vi "VISJS Viewer.vi"(4 "Extra Scripts":string, 5 "FileDependency In":map{path, T1}(c390), 6 "Options":string, 7 "OpenWebBrowser(False)":bool, 8 "error in":errorcluster, 9 "Embedd VISJS Librarya in HTMl File(False)":bool, 10 "HTMLFilePath":path, 11 "LibraryDependency":map{path, T3}(c390)) -> (0 "error out":errorcluster, 3 "HTMLFileContent":string)   [LabVIEW 2020, in "VISJS Viewer.lvlib"] (continued)
function(){if(\"undefined\"==typeof Reflect||!MT)return!1;if(MT.sham)return!1;if(\"function\"==typeof Proxy)return!0;try{return Boolean.prototype.valueOf.call(MT(Boolean,[],(function(){}))),!0}catch(g){return!1}}();return function(){var A,e=nb(g);if(t){var C=nb(this).constructor;A=MT(e,arguments,C)}else A=e.apply(this,arguments);return Ib(this,A)}}var NR=function(g){Cb(A,g);var t=DR(A);function A(g,e,C){return cn(this,A),t.call(this,g,e,C)}return kd(A,[{key:\"_line\",value:function(g,t,A){this._bezierCurve(g,t,A)}},{key:\"getViaNode\",value:function(){return this._getViaCoordinates()}},{key:\"_getViaCoordinates\",value:function(){var g,t,A=this.options.smooth.roundness,e=this.options.smooth.type,C=Math.abs(this.from.x-this.to.x),I=Math.abs(this.from.y-this.to.y);if(\"discrete\"===e||\"diagonalCross\"===e){var i,o;i=o=C<=I?A*I:A*C,this.from.x>this.to.x&&(i=-i),this.from.y>=this.to.y&&(o=-o);var n=this.from.x+i,r=this.from.y+o;return\"discrete\"===e&&(C<=I?n=C<A*I?this.from.x:n:r=I<A*C?this.from.y:r),{x:n,y:r}}if(\"straightCross\"===e){var s=(1-A)*C,a=(1-A)*I;return C<=I?(s=0,this.from.y<this.to.y&&(a=-a)):(this.from.x<this.to.x&&(s=-s),a=0),{x:this.to.x+s,y:this.to.y+a}}if(\"horizontal\"===e){var d=(1-A)*C;return this.from.x<this.to.x&&(d=-d),{x:this.to.x+d,y:this.from.y}}if(\"vertical\"===e){var h=(1-A)*I;return this.from.y<this.to.y&&(h=-h),{x:this.from.x,y:this.to.y+h}}if(\"curvedCW\"===e){C=this.to.x-this.from.x,I=this.from.y-this.to.y;var l=Math.sqrt(C*C+I*I),c=Math.PI,u=(Math.atan2(I,C)+(.5*A+.5)*c)%(2*c);return{x:this.from.x+(.5*A+.5)*l*Math.sin(u),y:this.from.y+(.5*A+.5)*l*Math.cos(u)}}if(\"curvedCCW\"===e){C=this.to.x-this.from.x,I=this.from.y-this.to.y;var p=Math.sqrt(C*C+I*I),f=Math.PI,v=(Math.atan2(I,C)+(.5*-A+.5)*f)%(2*f);return{x:this.from.x+(.5*A+.5)*p*Math.sin(v),y:this.from.y+(.5*A+.5)*p*Math.cos(v)}}g=t=C<=I?A*I:A*C,this.from.x>this.to.x&&(g=-g),this.from.y>=this.to.y&&(t=-t);var y=this.from.x+g,m=this.from.y+t;return C<=I?y=this.from.x<=this.to.x?this.to.x<y?this.to.x:y:this.to.x>y?this.to.x:y:m=this.from.y>=this.to.y?this.to.y>m?this.to.y:m:this.to.y<m?this.to.y:m,{x:y,y:m}}},{key:\"_findBorderPosition\",value:function(g,t){var A=arguments.length>2&&void 0!==arguments[2]?arguments[2]:{};return this._findBorderPositionBezier(g,t,A.via)}},{key:\"_getDistanceToEdge\",value:function(g,t,A,e,C,I){var i=arguments.length>6&&void 0!==arguments[6]?arguments[6]:this._getViaCoordinates();return this._getDistanceToBezierEdge(g,t,A,e,C,I,i)}},{key:\"getPoint\",value:function(g){var t=arguments.length>1&&void 0!==arguments[1]?arguments[1]:this._getViaCoordinates(),A=g;return{x:Math.pow(1-A,2)*this.fromPoint.x+2*A*(1-A)*t.x+Math.pow(A,2)*this.toPoint.x,y:Math.pow(1-A,2)*this.fromPoint.y+2*A*(1-A)*t.y+Math.pow(A,2)*this.toPoint.y}}}]),A}(ER);function RR(g){var t=function(){if(\"undefined\"==typeof Reflect||!MT)return!1;if(MT.sham)return!1;if(\"function\"==typeof Proxy)return!0;try{return Boolean.prototype.valueOf.call(MT(Boolean,[],(function(){}))),!0}catch(g){return!1}}();return function(){var A,e=nb(g);if(t){var C=nb(this).constructor;A=MT(e,arguments,C)}else A=e.apply(this,arguments);return Ib(this,A)}}var PR=function(g){Cb(A,g);var t=RR(A);function A(g,e,C){return cn(this,A),t.call(this,g,e,C)}return kd(A,[{key:\"_getDistanceToBezierEdge2\",value:function(g,t,A,e,C,I,i,o){for(var n=1e9,r=g,s=t,a=[0,0,0,0],d=1;d<10;d++){var h=.1*d;a[0]=Math.pow(1-h,3),a[1]=3*h*Math.pow(1-h,2),a[2]=3*Math.pow(h,2)*(1-h),a[3]=Math.pow(h,3);var l=a[0]*g+a[1]*i.x+a[2]*o.x+a[3]*A,c=a[0]*t+a[1]*i.y+a[2]*o.y+a[3]*e;if(d>0){var u=this._getDistanceToLine(r,s,l,c,C,I);n=u<n?u:n}r=l,s=c}return n}}]),A}(ER);function MR(g){var t=function(){if(\"undefined\"==typeof Reflect||!MT)return!1;if(MT.sham)return!1;if(\"function\"==typeof Proxy)return!0;try{return Boolean.prototype.valueOf.call(MT(Boolean,[],(function(){}))),!0}catch(g){return!1}}();return function(){var A,e=nb(g);if(t){var C=nb(this).constructor;A=MT(e,arguments,C)}else A=e.apply(this,arguments);return Ib(this,A)}}var BR=function(g){Cb(A,g);var t=MR(A);function A(g,e,C){return cn(this,A),t.call(this,g,e,C)}return kd(A,[{key:\"_line\",value:function(g,t,A){var e=A[0],C=A[1];this._bezierCurve(g,t,e,C)}},{key:\"_getViaCoordinates\",value:function(){var g,t,A,e,C=this.from.x-this.to.x,I=this.from.y-this.to.y,i=this.options.smooth.roundness;return(Math.abs(C)>Math.abs(I)||!0===this.options.smooth.forceDirection||\"horizontal\"===this.options.smooth.forceDirection)&&\"vertical\"!==this.options.smooth.forceDirection?(t=this.from.y,e=this.to.y,g=this.from.x-i*C,A=this.to.x+i*C):(t=this.from.y-i*I,e=this.to.y+i*I,g=this.from.x,A=this.to.x),[{x:g,y:t},{x:A,y:e}]}},{key:\"getViaNode\",value:function(){return this._getViaCoordinates()}},{key:\"_findBorderPosition\",value:function(g,t){return this._findBorderPositionBezier(g,t)}},{key:\"_getDistanceToEdge\",value:function(g,t,A,e,C,I){var i=lh(arguments.length>6&&void 0!==arguments[6]?arguments[6]:this._getViaCoordinates(),2),o=i[0],n=i[1];return this._getDistanceToBezierEdge2(g,t,A,e,C,I,o,n)}},{key:\"getPoint\",value:function(g){var t=lh(arguments.length>1&&void 0!==arguments[1]?arguments[1]:this._getViaCoordinates(),2),A=t[0],e=t[1],C=g,I=[Math.pow(1-C,3),3*C*Math.pow(1-C,2),3*Math.pow(C,2)*(1-C),Math.pow(C,3)];return{x:I[0]*this.fromPoint.x+I[1]*A.x+I[2]*e.x+I[3]*this.toPoint.x,y:I[0]*this.fromPoint.y+I[1]*A.y+I[2]*e.y+I[3]*this.toPoint.y}}}]),A}(PR);function zR(g){var t=function(){if(\"undefined\"==typeof Reflect||!MT)return!1;if(MT.sham)return!1;if(\"function\"==typeof Proxy)return!0;try{return Boolean.prototype.valueOf.call(MT(Boolean,[],(function(){}))),!0}catch(g){return!1}}();return function(){var A,e=nb(g);if(t){var C=nb(this).constructor;A=MT(e,arguments,C)}else A=e.apply(this,arguments);return Ib(this,A)}}var SR=function(g){Cb(A,g);var t=zR(A);function A(g,e,C){return cn(this,A),t.call(this,g,e,C)}return kd(A,[{key:\"_line\",value:function(g,t){g.beginPath(),g.moveTo(this.fromPoint.x,this.fromPoint.y),g.lineTo(this.toPoint.x,this.toPoint.y),this.enableShadow(g,t),g.stroke(),this.disableShadow(g,t)}},{key:\"getViaNode\",value:function(){}},{key:\"getPoint\",value:function(g){return{x:(1-g)*this.fromPoint.x+g*this.toPoint.x,y:(1-g)*this.fromPoint.y+g*this.toPoint.y}}},{key:\"_findBorderPosition\",value:function(g,t){var A=this.to,e=this.from;g.id===this.from.id&&(A=this.from,e=this.to);var C=Math.atan2(A.y-e.y,A.x-e.x),I=A.x-e.x,i=A.y-e.y,o=Math.sqrt(I*I+i*i),n=(o-g.distanceToBorder(t,C))/o;return{x:(1-n)*e.x+n*A.x,y:(1-n)*e.y+n*A.y,t:0}}},{key:\"_getDistanceToEdge\",value:function(g,t,A,e,C,I){return this._getDistanceToLine(g,t,A,e,C,I)}}]),A}(bR),ZR=function(){function g(t,A,e,C,I){if(cn(this,g),void 0===A)throw new Error(\"No body provided\");this.options=av(C),this.globalOptions=C,this.defaultOptions=I,this.body=A,this.imagelist=e,this.id=void 0,this.fromId=void 0,this.toId=void 0,this.selected=!1,this.hover=!1,this.labelDirty=!0,this.baseWidth=this.options.width,this.baseFontSize=this.options.font.size,this.from=void 0,this.to=void 0,this.edgeType=void 0,this.connected=!1,this.labelModule=new qD(this.body,this.options,!0),this.setOptions(t)}return kd(g,[{key:\"setOptions\",value:function(t){if(t){var A=void 0!==t.physics&&this.options.physics!==t.physics||void 0!==t.hidden&&(this.options.hidden||!1)!==(t.hidden||!1)||void 0!==t.from&&this.options.from!==t.from||void 0!==t.to&&this.options.to!==t.to;g.parseOptions(this.options,t,!0,this.globalOptions),void 0!==t.id&&(this.id=t.id),void 0!==t.from&&(this.fromId=t.from),void 0!==t.to&&(this.toId=t.to),void 0!==t.title&&(this.title=t.title),void 0!==t.value&&(t.value=SD(t.value));var e=[t,this.options,this.defaultOptions];return this.chooser=YD(\"edge\",e),this.updateLabelModule(t),A=this.updateEdgeType()||A,this._setInteractionWidths(),this.connect(),A}}},{key:\"getFormattingValues\",value:function(){var g=!0===this.options.arrows.to||!0===this.options.arrows.to.enabled,t=!0===this.options.arrows.from||!0===this.options.arrows.from.enabled,A=!0===this.options.arrows.middle||!0===this.options.arrows.middle.enabled,e=this.options.color.inherit,C={toArrow:g,toArrowScale:this.options.arrows.to.scaleFactor,toArrowType:this.options.arrows.to.type,toArrowSrc:this.options.arrows.to.src,toArrowImageWidth:this.options.arrows.to.imageWidth,toArrowImageHeight:this.options.arrows.to.imageHeight,middleArrow:A,middleArrowScale:this.options.arrows.middle.scaleFactor,middleArrowType:this.options.arrows.middle.type,middleArrowSrc:this.options.arrows.middle.src,middleArrowImageWidth:this.options.arrows.middle.imageWidth,middleArrowImageHeight:this.options.arrows.middle.imageHeight,fromArrow:t,fromArrowScale:this.options.arrows.from.scaleFactor,fromArrowType:this.options.arrows.from.type,fromArrowSrc:this.options.arrows.from.src,fromArrowImageWidth:this.options.arrows.from.imageWidth,fromArrowImageHeight:this.options.arrows.from.imageHeight,arrowStrikethrough:this.options.arrowStrikethrough,color:e?void 0:this.options.color.color,inheritsColor:e,opacity:this.options.color.opacity,hidden:this.options.hidden,length:this.options.length,shadow:this.options.shadow.enabled,shadowColor:this.options.shadow.color,shadowSize:this.options.shadow.size,shadowX:this.options.shadow.x,shadowY:this.options.shadow.y,dashes:this.options.dashes,width:this.options.width,background:this.options.background.enabled,backgroundColor:this.options.background.color,backgroundSize:this.options.background.size,backgroundDashes:this.options.background.dashes};if(this.selected||this.hover)if(!0===this.chooser){if(this.selected){var I=this.options.selectionWidth;\"function\"==typeof I?C.width=I(C.width):\"number\"==typeof I&&(C.width+=I),C.width=Math.max(C.width,.3/this.body.view.scale),C.color=this.options.color.highlight,C.shadow=this.options.shadow.enabled}else if(this.hover){var i=this.options.hoverWidth;\"function\"==typeof i?C.width=i(C.width):\"number\"==typeof i&&(C.width+=i),C.width=Math.max(C.width,.3/this.body.view.scale),C.color=this.options.color.hover,C.shadow=this.options.shadow.enabled}}else\"function\"==typeof this.chooser&&(this.chooser(C,this.options.id,this.selected,this.hover),void 0!==C.color&&(C.inheritsColor=!1),!1===C.shadow&&(C.shadowColor===this.options.shadow.color&&C.shadowSize===this.options.shadow.size&&C.shadowX===this.options.shadow.x&&C.shadowY===this.options.shadow.y||(C.shadow=!0)));else C.shadow=this.options.shadow.enabled,C.width=Math.max(C.width,.3/this.body.view.scale);return C}},{key:\"updateLabelModule\",value:function(g){var t=[g,this.options,this.globalOptions,this.defaultOptions];this.labelModule.update(this.options,t),void 0!==this.labelModule.baseSize&&(this.baseFontSize=this.labelModule.baseSize)}},{key:\"updateEdgeType\",value:function(){var g=this.options.smooth,t=!1,A=!0;return void 0!==this.edgeType&&((this.edgeType instanceof TR&&!0===g.enabled&&\"dynamic\"===g.type||this.edgeType instanceof BR&&!0===g.enabled&&\"cubicBezier\"===g.type||this.edgeType instanceof NR&&!0===g.enabled&&\"dynamic\"!==g.type&&\"cubicBezier\"!==g.type||this.edgeType instanceof SR&&!1===g.type.enabled)&&(A=!1),!0===A&&(t=this.cleanup())),!0===A?!0===g.enabled?\"dynamic\"===g.type?(t=!0,this.edgeType=new TR(this.options,this.body,this.labelModule)):\"cubicBezier\"===g.type?this.edgeType=new BR(this.options,this.body,this.labelModule):this.edgeType=new NR(this.options,this.body,this.labelModule):this.edgeType=new SR(this.options,this.body,this.labelModule):this.edgeType.setOptions(this.options),t}},{key:\"connect\",value:function(){this.disconnect(),this.from=this.body.nodes[this.fromId]||void 0,this.to=this.body.nodes[this.toId]||void 0,this.connected=void 0!==this.from&&void 0!==this.to,!0===this.connected?(this.from.attachEdge(this),this.to.attachEdge(this)):(this.from&&this.from.detachEdge(this),this.to&&this.to.detachEdge(this)),this.edgeType.connect()}},{key:\"disconnect\",value:function(){this.from&&(this.from.detachEdge(this),this.from=void 0),this.to&&(this.to.detachEdge(this),this.to=void 0),this.connected=!1}},{key:\"getTitle\",value:function(){return this.title}},{key:\"isSelected\",value:function(){return this.selected}},{key:\"getValue\",value:function(){return this.options.value}},{key:\"setValueRange\",value:function(g,t,A){if(void 0!==this.options.value){var e=this.options.scaling.customScalingFunction(g,t,A,this.options.value),C=this.options.scaling.max-this.options.scaling.min;if(!0===this.options.scaling.label.enabled){var I=this.options.scaling.label.max-this.options.scaling.label.min;this.options.font.size=this.options.scaling.label.min+e*I}this.options.width=this.options.scaling.min+e*C}else this.options.width=this.baseWidth,this.options.font.size=this.baseFontSize;this._setInteractionWidths(),this.updateLabelModule()}},{key:\"_setInteractionWidths\",value:function(){\"function\"==typeof this.options.hoverWidth?this.edgeType.hoverWidth=this.options.hoverWidth(this.options.width):this.edgeType.hoverWidth=this.options.hoverWidth+this.options.width,\"function\"==typeof this.options.selectionWidth?this.edgeType.selectionWidth=this.options.selectionWidth(this.options.width):this.edgeType.selectionWidth=this.options.selectionWidth+this.options.width}},{key:\"draw\",value:function(g){var t=this.getFormattingValues();if(!t.hidden){var A=this.edgeType.getViaNode();this.edgeType.drawLine(g,t,this.selected,this.hover,A),this.drawLabel(g,A)}}},{key:\"drawArrows\",value:function(g){var t=this.getFormattingValues();if(!t.hidden){var A=this.edgeType.getViaNode(),e={};this.edgeType.fromPoint=this.edgeType.from,this.edgeType.toPoint=this.edgeType.to,t.fromArrow&&(e.from=this.edgeType.getArrowData(g,\"from\",A,this.selected,this.hover,t),!1===t.arrowStrikethrough&&(this.edgeType.fromPoint=e.from.core),t.fromArrowSrc&&(e.from.image=this.imagelist.load(t.fromArrowSrc)),t.fromArrowImageWidth&&(e.from.imageWidth=t.fromArrowImageWidth),t.fromArrowImageHeight&&(e.from.imageHeight=t.fromArrowImageHeight)),t.toArrow&&(e.to=this.edgeType.getArrowData(g,\"to\",A,this.selected,this.hover,t),!1===t.arrowStrikethrough&&(this.edgeType.toPoint=e.to.core),t.toArrowSrc&&(e.to.image=this.imagelist.load(t.toArrowSrc)),t.toArrowImageWidth&&(e.to.imageWidth=t.toArrowImageWidth),t.toArrowImageHeight&&(e.to.imageHeight=t.toArrowImageHeight)),t.middleArrow&&(e.middle=this.edgeType.getArrowData(g,\"middle\",A,this.selected,this.hover,t),t.middleArrowSrc&&(e.middle.image=this.imagelist.load(t.middleArrowSrc)),t.middleArrowImageWidth&&(e.middle.imageWidth=t.middleArrowImageWidth),t.middleArrowImageHeight&&(e.middle.imageHeight=t.middleArrowImageHeight)),t.fromArrow&&this.edgeType.drawArrowHead(g,t,this.selected,this.hover,e.from),t.middleArrow&&this.edgeType.drawArrowHead(g,t,this.selected,this.hover,e.middle),t.toArrow&&this.edgeType.drawArrowHead(g,t,this.selected,this.hover,e.to)}}},{key:\"drawLabel\",value:function(g,t){if(void 0!==this.options.label){var A,e=this.from,C=this.to;if(this.labelModule.differentState(this.selected,this.hover)&&this.labelModule.getTextSize(g,this.selected,this.hover),e.id!=C.id){this.labelModule.pointToSelf=!1,A=this.edgeType.getPoint(.5,t),g.save();var I=this._getRotation(g);0!=I.angle&&(g.translate(I.x,I.y),g.rotate(I.angle)),this.labelModule.draw(g,A.x,A.y,this.selected,this.hover),g.restore()}else{this.labelModule.pointToSelf=!0;var i=UD(g,this.options.selfReference.angle,this.options.selfReference.size,e);A=this._pointOnCircle(i.x,i.y,this.options.selfReference.size,this.options.selfReference.angle),this.labelModule.draw(g,A.x,A.y,this.selected,this.hover)}}}},{key:\"getItemsOnPoint\",value:function(g){var t=[];if(this.labelModule.visible()){var A=this._getRotation();WD(this.labelModule.getSize(),g,A)&&t.push({edgeId:this.id,labelId:0})}var e={left:g.x,top:g.y};return this.isOverlappingWith(e)&&t.push({edgeId:this.id}),t}},{key:\"isOverlappingWith\",value:function(g){if(this.connected){var t=this.from.x,A=this.from.y,e=this.to.x,C=this.to.y,I=g.left,i=g.top;return this.edgeType.getDistanceToEdge(t,A,e,C,I,i)<10}return!1}},{key:\"_getRotation\",value:function(g){var t=this.edgeType.getViaNode(),A=this.edgeType.getPoint(.5,t);void 0!==g&&this.labelModule.calculateLabelSize(g,this.selected,this.hover,A.x,A.y);var e={x:A.x,y:this.labelModule.size.yLine,angle:0};if(!this.labelModule.visible())return e;if(\"horizontal\"===this.options.font.align)return e;var C=this.from.y-this.to.y,I=this.from.x-this.to.x,i=Math.atan2(C,I);return(i<-1&&I<0||i>0&&I<0)&&(i+=Math.PI),e.angle=i,e}},{key:\"_pointOnCircle\",value:function(g,t,A,e){return{x:g+A*Math.cos(e),y:t-A*Math.sin(e)}}},{key:\"select\",value:function(){this.selected=!0}},{key:\"unselect\",value:function(){this.selected=!1}},{key:\"cleanup\",value:function(){return this.edgeType.cleanup()}},{key:\"remove\",value:function(){this.cleanup(),this.disconnect(),delete this.body.edges[this.id]}},{key:\"endPointsValid\",value:function(){return void 0!==this.body.nodes[this.fromId]&&void 0!==this.body.nodes[this.toId]}}],[{key:\"parseOptions\",value:function(g,t){var A=arguments.length>2&&void 0!==arguments[2]&&arguments[2],e=arguments.length>3&&void 0!==arguments[3]?arguments[3]:{},C=arguments.length>4&&void 0!==arguments[4]&&arguments[4];if(Xf([\"endPointOffset\",\"arrowStrikethrough\",\"id\",\"from\",\"hidden\",\"hoverWidth\",\"labelHighlightBold\",\"length\",\"line\",\"opacity\",\"physics\",\"scaling\",\"selectionWidth\",\"selfReferenceSize\",\"selfReference\",\"to\",\"title\",\"value\",\"width\",\"font\",\"chosen\",\"widthConstraint\"],g,t,A),void 0!==t.endPointOffset&&void 0!==t.endPointOffset.from&&(Ym(t.endPointOffset.from)?g.endPointOffset.from=t.endPointOffset.from:(g.endPointOffset.from=void 0!==e.endPointOffset.from?e.endPointOffset.from:0,console.error(\"endPointOffset.from is not a valid number\"))),void 0!==t.endPointOffset&&void 0!==t.endPointOffset.to&&(Ym(t.endPointOffset.to)?g.endPointOffset.to=t.endPointOffset.to:(g.endPointOffset.to=void 0!==e.endPointOffset.to?e.endPointOffset.to:0,console.error(\"endPointOffset.to is not a valid number\"))),QD(t.label)?g.label=t.label:QD(g.label)||(g.label=void 0),dv(g,t,\"smooth\",e),dv(g,t,\"shadow\",e),dv(g,t,\"background\",e),void 0!==t.dashes&&null!==t.dashes?g.dashes=t.dashes:!0===A&&null===t.dashes&&(g.dashes=$c(e.dashes)),void 0!==t.scaling&&null!==t.scaling?(void 0!==t.scaling.min&&(g.scaling.min=t.scaling.min),void 0!==t.scaling.max&&(g.scaling.max=t.scaling.max),dv(g.scaling,t.scaling,\"label\",e.scaling)):!0===A&&null===t.scaling&&(g.scaling=$c(e.scaling)),void 0!==t.arrows&&null!==t.arrows)if(\"string\"==typeof t.arrows){var I=t.arrows.toLowerCase();g.arrows.to.enabled=-1!=Xc(I).call(I,\"to\"),g.arrows.middle.enabled=-1!=Xc(I).call(I,\"middle\"),g.arrows.from.enabled=-1!=Xc(I).call(I,\"from\")}else{if(\"object\"!==yd(t.arrows))throw new Error(\"The arrow newOptions can only be an object or a string. Refer to the documentation. You used:\"+eu(t.arrows));dv(g.arrows,t.arrows,\"to\",e.arrows),dv(g.arrows,t.arrows,\"middle\",e.arrows),dv(g.arrows,t.arrows,\"from\",e.arrows)}else!0===A&&null===t.arrows&&(g.arrows=$c(e.arrows));if(void 0!==t.color&&null!==t.color){var i=Uf(t.color)?{color:t.color,highlight:t.color,hover:t.color,inherit:!1,opacity:1}:t.color,o=g.color;if(C)qf(o,e.color,!1,A);else for(var n in o)Object.prototype.hasOwnProperty.call(o,n)&&delete o[n];if(Uf(o))o.color=o,o.highlight=o,o.hover=o,o.inherit=!1,void 0===i.opacity&&(o.opacity=1);else{var r=!1;void 0!==i.color&&(o.color=i.color,r=!0),void 0!==i.highlight&&(o.highlight=i.highlight,r=!0),void 0!==i.hover&&(o.hover=i.hover,r=!0),void 0!==i.inherit&&(o.inherit=i.inherit),void 0!==i.opacity&&(o.opacity=Math.min(1,Math.max(0,i.opacity))),!0===r?o.inherit=!1:void 0===o.inherit&&(o.inherit=\"from\")}}else!0===A&&null===t.color&&(g.color=av(e.color));!0===A&&null===t.font&&(g.font=av(e.font)),Object.prototype.hasOwnProperty.call(t,\"selfReferenceSize\")&&(console.warn(\"The selfReferenceSize property has been deprecated. Please use 
